vi "LabVIEW Time to FPGA Time.vi"(1 "LabVIEW time":timestamp format="%<%.9X\n%x>T") -> (0 "FPGA time (ns)":u64 format="%.2f")   [LabVIEW 2013, in "FPGA Timekeeper.lvlib"]
doc: "Converts LabVIEW Time into FPGA Time. Note that the FPGA Timekeeper keeps time in nanoseconds starting from January 1st, 1970."
uses:
  FPGA Timekeeper.lvlib
panel:
  out "fixed-point":fxp<+/-,64,44> format="%#_25g"
  out "conversion":i64
  out "double precision float 3":dbl format="%#_22g"
  out "integer":i64
  out "double precision float 2":dbl format="%_22g"
  out "double precision float":dbl format="%_24g"
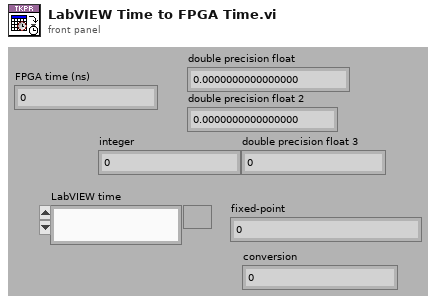
[diagram p1: front panel]
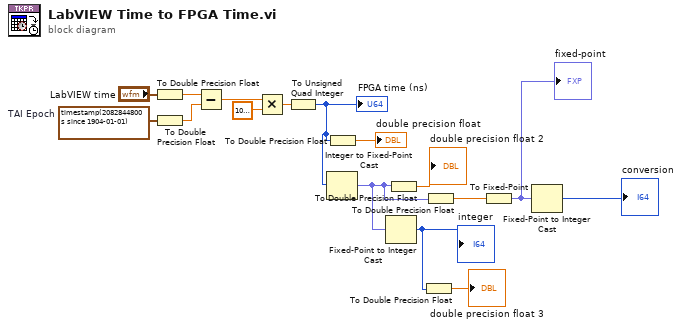
[diagram p0: block diagram]
diagram:
  w16 = timestamp(2082844800 s since 1904-01-01)  # TAI Epoch
  n1 = To Double Precision Float(number="LabVIEW time") -> (double precision float=w13:dbl)
  n2 = To Double Precision Float(number=w16) -> (double precision float=w12:dbl)
  n3 = Subtract(x=w13, y=w12) -> (x-y=w11:dbl)
  n4 = Multiply(x=w11, y=1000000000.0) -> (x*y=w10:dbl)
  n5 = To Unsigned Quad Integer(1:w10) -> (0:w8:u64)
  "FPGA time (ns)" <- w8
  n6 = Integer to Fixed-Point Cast(integer=w8) -> (fixed-point=w4:fxp<+/-,64,44>)  [unwired: 1 in]
  n7 = To Double Precision Float(number=w8) -> (double precision float=→"double precision float":dbl)
  n8 = Fixed-Point to Integer Cast(1:w4) -> (0:w6:i64)
  "integer" <- w6
  n9 = To Double Precision Float(number=w4) -> (double precision float=→"double precision float 2":dbl)
  n10 = To Double Precision Float(number=w6) -> (double precision float=→"double precision float 3":dbl)
  n11 = To Double Precision Float(number=w4) -> (double precision float=w3:dbl)
  n12 = To Fixed-Point(number=w3) -> (fixed-point=w2:fxp<+/-,64,44>)  [unwired: 1 in]
  "fixed-point" <- w2
  n13 = Fixed-Point to Integer Cast(1:w2) -> (0:→"conversion":i64)
